vi "Write broker.vi"(8 "error in (no error)":errorcluster, 10 "broker":T1, 11 "MQTT Client in":refnum<class "MQTT Client.lvclass">) -> (0 "error out":errorcluster, 3 "MQTT Client out":refnum<class "MQTT Client.lvclass">)   [LabVIEW 2020, in "MQTT Client.lvclass"]
uses:
  MQTT Client.lvclass
  mqttTypedef/ConnectionConfig.ctl
  MQTT Client.lvclass/MQTT Client.ctl
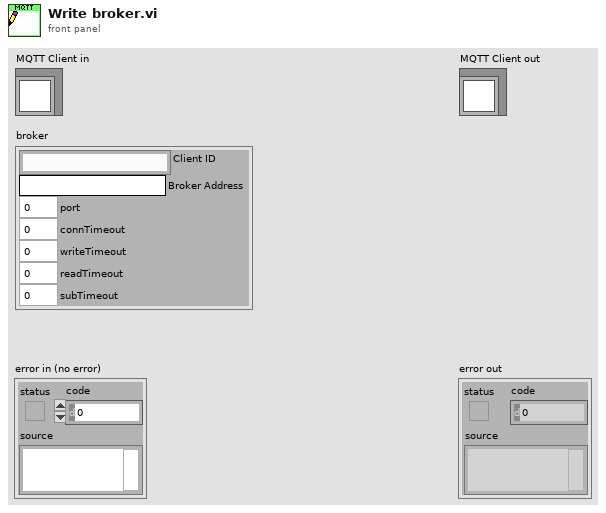
[diagram p1: front panel]
types:
  T1 = typedef "MQTT Client.lvclass/ConnectionConfig.ctl" = cluster{"Client ID":string, "Broker Address":string, "port":u16, "connTimeout":i32, "writeTimeout":i32, "readTimeout":i32, "subTimeout":i32}
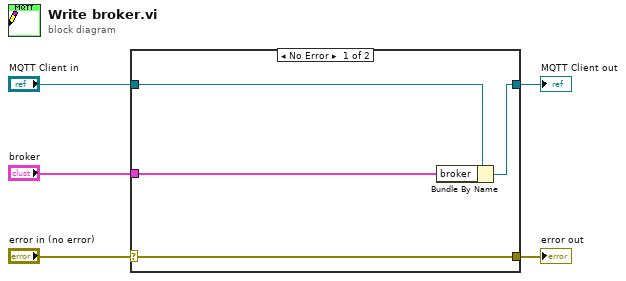
[diagram p0: block diagram]
diagram:
  n1 = case shown="No Error" "error in (no error)" {
    selector: "error in (no error)" -> [w9 w10]
    tunnel: [w9 w10] -> w4
    tunnel: [w7 w11] -> w2
    tunnel: "MQTT Client in" -> [w8 w11]
    tunnel: "broker" -> [w6 _]
    frame No Error {
      n2 = Bundle By Name(cluster=w8, "broker"=w6) -> (w7:refnum<class "MQTT Client.lvclass">)
    }
    frame Error {
    }
  }
  "error out" <- w4
  "MQTT Client out" <- w2
